vi "New Analog Writer.vi"(8 "error in (no error)":errorcluster, 10 "DAQmx Task":refnum<k21>, 11 "Analog Writer in":refnum<class "Analog Writer.lvclass">) -> (0 "error out":errorcluster, 3 "Analog Writer out":refnum<class "Analog Writer.lvclass">)   [LabVIEW 2024, in "DAQmx Actor.lvlib" / "Analog Writer.lvclass"]
uses:
  Analog Writer.lvclass
  Analog Writer.lvclass/Analog Writer.ctl
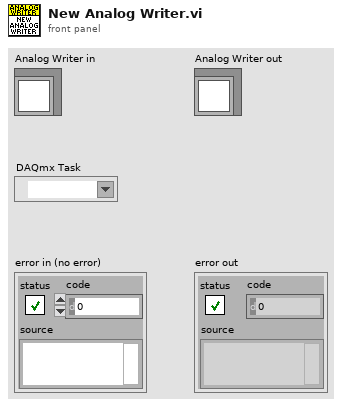
[diagram p1: front panel]
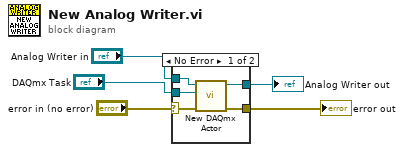
[diagram p0: block diagram]
diagram:
  n1 = case shown="No Error" "error in (no error)" {
    selector: "error in (no error)" -> [w7 w12]
    tunnel: [w6 w12] -> w4
    tunnel: [w9 w11] -> w2
    tunnel: "Analog Writer in" -> [w10 w11]
    tunnel: "DAQmx Task" -> [w8 _]
    frame No Error {
      n2 = call-dynamic "New DAQmx Actor.vi"("error in (no error)"=w7, "DAQmx Task"=w8, "DAQmx Actor in"=w10) -> ("error out"=w6:errorcluster, "DAQmx Actor out"=w9:refnum<class "Analog Writer.lvclass">)  [unwired: 7 in]
    }
    frame Error {
    }
  }
  "error out" <- w4
  "Analog Writer out" <- w2
